vi "U16-I32.vi"(11 "数组":u8[](array[numeric])=[255, 254, 252]) -> (3 "I32转换":i16)   [LabVIEW 2012]
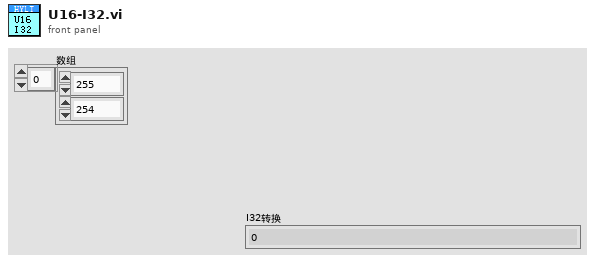
[diagram p1: front panel]
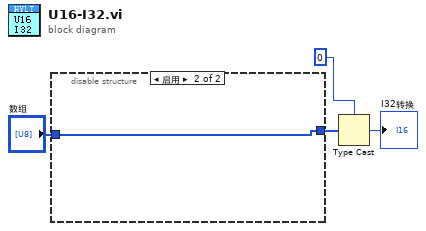
[diagram p0: block diagram]
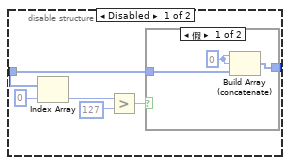
[diagram p2: hidden frame]
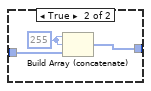
[diagram p3: hidden frame]
diagram:
  n1 = disable-structure shown="启用" {
    disable-tunnel: [w6 w17] -> w3
    disable-tunnel: "数组" -> [w5 w17]
    frame Disabled {
      n2 = Index Array(array=w5, index=0 ("索引")) -> (element=w9:u8)
      n3 = Greater?(x=w9, y=u8 127) -> (0:w7:bool)
      n4 = case shown="假" w7 {
        tunnel: w5 -> [w13 w16]
        tunnel: [w12 w15] -> w6
        frame False {
          w11 = u8 0 ("y")
          n5 = Build Array (concatenate)(w11, w11, w13) -> (w12:u8[])
        }
        frame True {
          w14 = u8 255 ("y")
          n6 = Build Array (concatenate)(w14, w14, w16) -> (w15:u8[])
        }
      }
    }
    frame Enabled {
    }
  }
  n7 = Type Cast(type=i16 0, x=w3) -> (*(type *) &x=→"I32转换":i16)
